vi "PanelWizard_Facade.vi"(0 "Data In":T6, 2 "Display State In":T2={"DisplayStyle"=enum."3D Style", "LaunchType"=enum."LaunchHDV", "UserVIPath"=path "", "Button Text"="", "UseDefaultButtonText?"=TRUE, "Run User VI?"=TRUE, "CommandLine"="", "StandardInput"="", "Working Directory"=path ""}, 3 "Container State":T5) -> (6 "Data Out":T6, 7 "Display State Out":T2={"DisplayStyle"=enum."3D Style", "LaunchType"=enum."LaunchHDV", "UserVIPath"=path "", "Button Text"="", "UseDefaultButtonText?"=TRUE, "Run User VI?"=TRUE, "CommandLine"="", "StandardInput"="", "Working Directory"=path ""}, 8 "Action":T1)   [LabVIEW 2012, in "PanelWizard.xctl"]
uses:
  PanelWizard.xctl
  PanelWizard_Data.ctl
  <vilib>/_xctls/Container State.ctl
  PanelWizard_State.ctl
  PanelWizard_DisplayType.ctl
  PanelWizard_LaunchOptions.ctl
  <vilib>/_xctls/Action.ctl
  <vilib>/_xctls/XControlSupport.lvlib
  <vilib>/lvdsc/NI_DSC.lvlib
panel:
  in  "RoundStyle":bool
  in  "SystemButton":bool
  in  "3dButton":bool
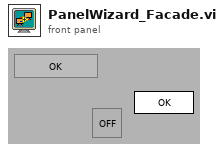
[diagram p1: front panel]
types:
  T1 = typedef "XControlSupport.lvlib/Action.ctl" = cluster{"Data Changed?":bool, "State Changed?":bool, "Action Name":string}
  T2 = typedef "PanelWizard.xctl/PanelWizard_State.ctl" = cluster{"DisplayStyle":T3, "LaunchType":T4, "UserVIPath":path, "Button Text":string, "UseDefaultButtonText?":bool, "Run User VI?":bool, "CommandLine":string, "StandardInput":string, "Working Directory":path}
  T3 = typedef "PanelWizard.xctl/PanelWizard_DisplayType.ctl" = enum16{"3D Style", "LabVIEW Classic Style", "System Style"}
  T4 = typedef "PanelWizard.xctl/PanelWizard_LaunchOptions.ctl" = enum16{"LaunchHDV", "LaunchSVMonitor", "LaunchUserVI", "Run command line"}
  T5 = typedef "XControlSupport.lvlib/Container State.ctl" = cluster{"Indicator?":bool, "Run Mode?":bool, " Refnum":refnum<vi>}
  T6 = typedef "PanelWizard.xctl/PanelWizard_Data.ctl" = bool
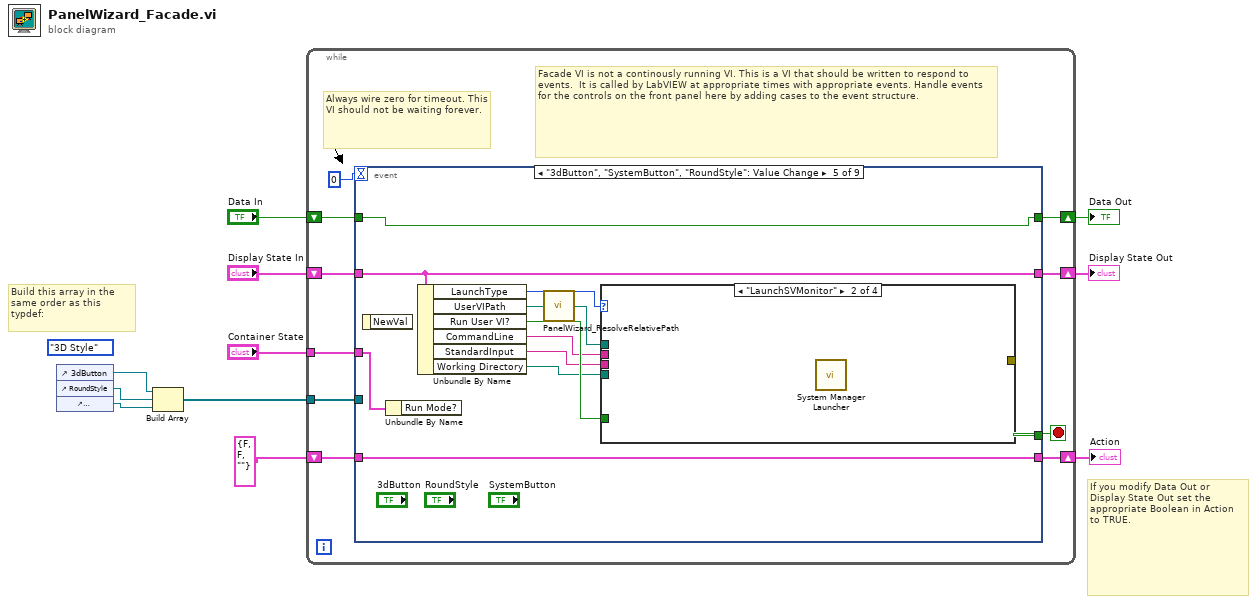
[diagram p0: block diagram]
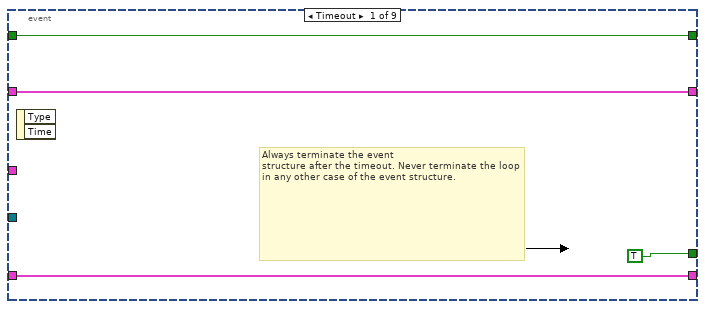
[diagram p2: hidden frame]
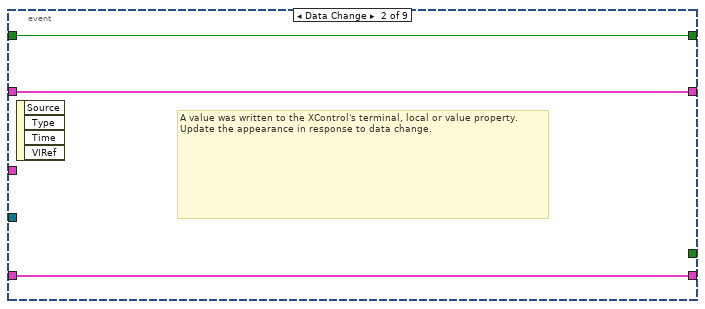
[diagram p3: hidden frame]
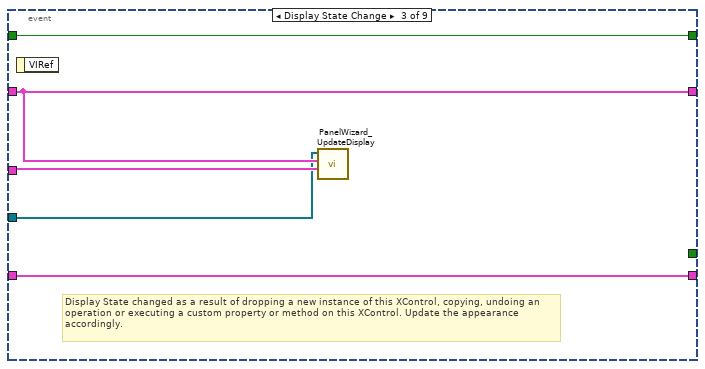
[diagram p4: hidden frame]
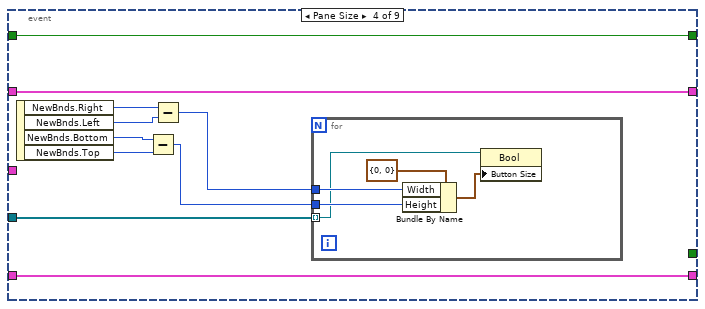
[diagram p5: hidden frame]
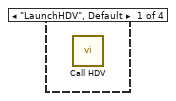
[diagram p6: hidden frame]
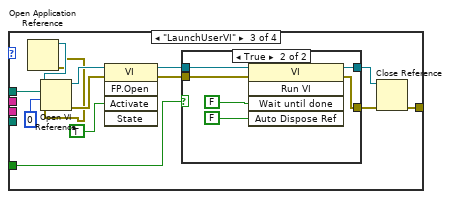
[diagram p7: hidden frame]
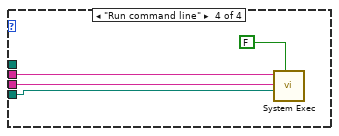
[diagram p9: hidden frame]
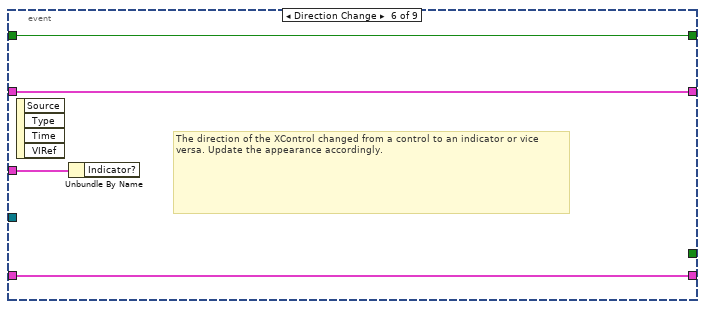
[diagram p10: hidden frame]
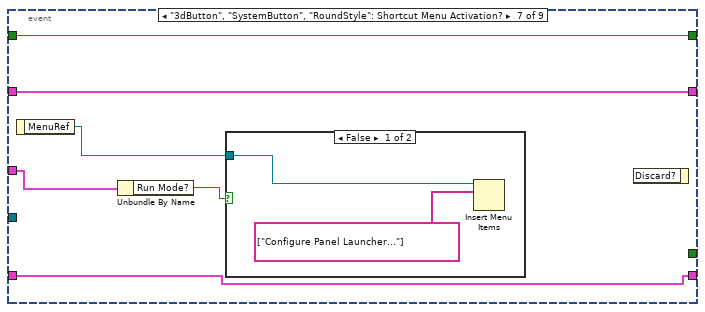
[diagram p11: hidden frame]
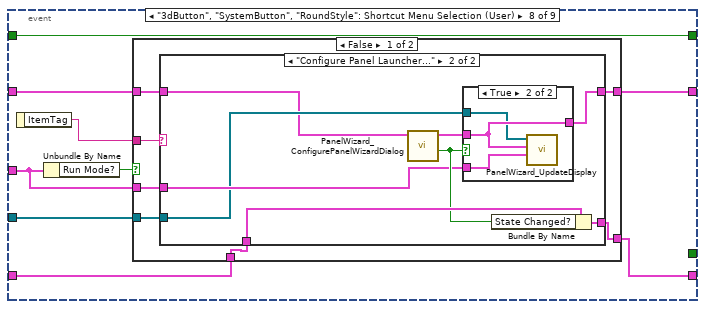
[diagram p13: hidden frame]
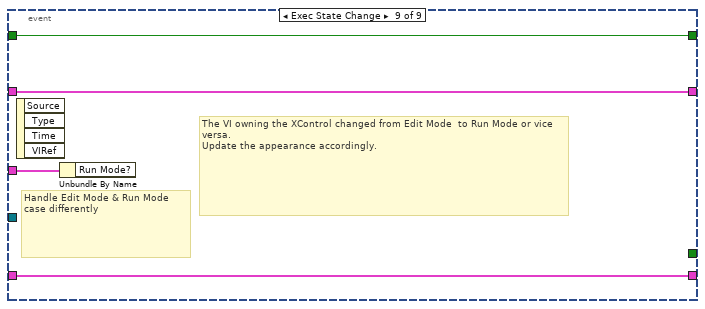
[diagram p17: hidden frame]
diagram:
  (unwired) PanelWizard_DisplayType."3D Style" ("PanelWizard_DisplayTypes")
  # "Build this array in the same order as this typdef:"
  # "If you modify Data Out or\nDisplay State Out set the\nappropriate Boolean in Action\nto TRUE."
  n1 = control-ref of="3dButton"() -> (w4:refnum<vi>)
  n2 = control-ref of="RoundStyle"() -> (w3:refnum<vi>)
  n3 = control-ref of="SystemButton"() -> (w2:refnum<vi>)
  n4 = Build Array(w4, w3, w2) -> (w1:refnum<vi>[])
  n5 = while {
    shift-right: [w20] -> w8
    shift-left: "Display State In" -> [w21]
    tunnel: "Container State" -> [w17]
    shift-right: [w15] -> w11
    shift-left: "Data In" -> [w16]
    shift-right: [w13] -> w6
    shift-left: T1 {"Data Changed?"=FALSE, "State Changed?"=FALSE, "Action Name"=""} ("Action") -> [w14]
    tunnel: w1 -> [w12]
    stop <- w19 stop-if-true
    # "Facade VI is not a continously running VI. This is a VI that should be written to respond to events.  It is called by LabVIEW at appropriate times with appropriate events. Handle events for the controls on the front panel here by adding cases to the event structure."
    # "Always wire zero for timeout. This\nVI should not be waiting forever."
    n6 = event shown="[4] \"3dButton\", \"SystemButton\", \"RoundStyle\": Value Change" {
      selector: _ -> [_ _ _ _ _ _ _ _ _]
      dyn-events: _ -> [_ _ _ _ _ _ _ _ _]
      timeout: 0 -> [_ _ _ _ _ _ _ _ _]
      tunnel: w21 -> [w23 w27 w30 w35 w57 w87 w91 w103 w131]
      tunnel: [w23 w27 w30 w35 w57 w87 w91 w102 w131] -> w20
      tunnel: [TRUE _ _ _ _ _ _ _ _] -> w19
      tunnel: w17 -> [_ _ w31 _ w55 w88 w92 w97 w132]
      tunnel: w16 -> [w22 w28 w33 w36 w56 w86 w89 w105 w130]
      tunnel: [w22 w28 w33 w36 w56 w86 w89 w105 w130] -> w15
      tunnel: [w24 w26 w32 w43 w58 w85 w90 w100 w129] -> w13
      tunnel: w14 -> [w24 w26 w32 w43 w58 w85 w90 w101 w129]
      tunnel: w12 -> [_ _ w29 w34 _ _ _ w98 _]
      event Timeout {
        # "Always terminate the event\nstructure after the timeout. Never terminate the loop in any other case of the event structure."
        n7 = event-data() -> ()  [unwired: 1 in, 2 out]
      }
      event Data Change {
        # "A value was written to the XControl's terminal, local or value property.\nUpdate the appearance in response to data change."
        n8 = event-data() -> ()  [unwired: 1 in, 4 out]
      }
      event Display State Change {
        # "Display State changed as a result of dropping a new instance of this XControl, copying, undoing an operation or executing a custom property or method on this XControl. Update the appearance accordingly."
        n9 = event-data() -> ()  [unwired: 1 in, 1 out]
        n10 = call "PanelWizard_UpdateDisplay.vi"("Container State"=w31, "Display State In"=w30, "Button Refs"=w29) -> ()  [unwired: 9 in]
      }
      event Pane Size {
        n11 = event-data() -> ("NewBnds.Right"=w42:i16, "NewBnds.Left"=w41:i16, "NewBnds.Bottom"=w40:i16, "NewBnds.Top"=w39:i16)  [unwired: 1 in]
        n12 = Subtract(x=w40, y=w39) -> (x-y=w37:i16)
        n13 = Subtract(x=w42, y=w41) -> (x-y=w38:i16)
        n14 = for {
          tunnel: w38 -> [w47]
          tunnel: w37 -> [w46]
          tunnel: w34 -> [w44] mode=indexing
          n15 = Bundle By Name(cluster=cluster{"Width":u32, "Height":u32} {"Width"=0, "Height"=0} ("Button Size"), "Width"=w47, "Height"=w46) -> (w45:cluster{"Width":u32, "Height":u32})
          n16 = property class="Bool"(reference=w44, "Button Size"=w45) -> ()  [unwired: 1 in, 2 out]
        }
      }
      event "3dButton", "SystemButton", "RoundStyle": Value Change {
        n17 = event-data() -> ()  [unwired: 1 in, 1 out]
        n18 = Unbundle By Name(w55) -> ()  [unwired: 1 out]
        n19 = Unbundle By Name(w57) -> ("LaunchType"=w59:T4, "UserVIPath"=w50:path, "Run User VI?"=w54:bool, "CommandLine"=w53:string, "StandardInput"=w52:string, "Working Directory"=w51:path)
        n20 = call "PanelWizard_ResolveRelativePath.vi"("Relative Path"=w50) -> ("Absolute  Path"=w49:path)
        n21 = case shown="\"LaunchSVMonitor\"" w59 {
          tunnel: w49 -> [_ _ w72 _]
          tunnel: [_ _ w68 _] -> _
          tunnel: w54 -> [_ _ w62 _]
          tunnel: w53 -> [_ _ _ w83]
          tunnel: w52 -> [_ _ _ w82]
          tunnel: w51 -> [_ _ _ w81]
          frame "LaunchHDV", Default {
            n22 = call <vilib>:"Call HDV.vi"() -> ()  [unwired: 14 in, 2 out]
          }
          frame "LaunchSVMonitor" {
            n23 = call "System Manager Launcher.vi"() -> ()  [unwired: 2 in]
          }
          frame "LaunchUserVI" {
            n24 = Open Application Reference() -> (0:w60:errorcluster, 3:w61:refnum<vi>)  [unwired: 4 in]
            n25 = Open VI Reference(application reference (local)=w61, vi path=w72, options=0, error in (no error)=w60) -> (vi reference=w67:refnum<vi>, error out=w64:errorcluster)  [unwired: 2 in]
            n26 = invoke class="VI" method="FP.Open"(reference=w67, error in=w64, "Activate"=TRUE ("Activate?")) -> (reference out=w66:refnum<vi>, error out=w65:errorcluster)  [unwired: 2 in, 3 out]
            n27 = case shown="True" w62 {
              tunnel: [w74 w80] -> w70
              tunnel: [w73 w79] -> w69
              tunnel: w66 -> [w74 w78]
              tunnel: w65 -> [w73 w77]
              frame False {
              }
              frame True {
                n28 = invoke class="VI" method="Run VI"(reference=w78, error in=w77, "Wait until done"=FALSE ("Wait Until Done"), "Auto Dispose Ref"=FALSE ("Wait Until Done")) -> (reference out=w80:refnum<vi>, error out=w79:errorcluster)  [unwired: 1 in, 3 out]
              }
            }
            n29 = Close Reference(reference=w70, error in (no error)=w69) -> (error out=w68:errorcluster)
          }
          frame "Run command line" {
            n30 = call <vilib>:"System Exec.vi"("wait until completion? (T)"=FALSE, "working directory"=w81, "standard input"=w82, "command line"=w83) -> ()  [unwired: 4 in, 4 out]
          }
        }
      }
      event Direction Change {
        # "The direction of the XControl changed from a control to an indicator or vice versa. Update the appearance accordingly."
        n31 = event-data() -> ()  [unwired: 1 in, 4 out]
        n32 = Unbundle By Name(w88) -> ()  [unwired: 1 out]
      }
      event "3dButton", "SystemButton", "RoundStyle": Shortcut Menu Activation? {
        n33 = event-data() -> ("MenuRef"=w93:refnum<k9>)  [unwired: 1 in]
        n34 = Unbundle By Name(w92) -> ("Run Mode?"=w94:bool)
        n35 = case shown="False" w94 {
          tunnel: w93 -> [w96 _]
          frame False {
            n36 = Insert Menu Items(8:string[] ["Configure Panel Launcher..."] ("item names"), 9:w96) -> ()  [unwired: 4 in, 3 out]
          }
          frame True {
          }
        }
        n37 = event-data() -> ()  [unwired: 2 in, 1 out]
      }
      event "3dButton", "SystemButton", "RoundStyle": Shortcut Menu Selection (User) {
        n38 = event-data() -> ("ItemTag"=w99:string)  [unwired: 1 in]
        n39 = Unbundle By Name(w97) -> ("Run Mode?"=w104:bool)
        n40 = case shown="False" w104 {
          tunnel: w99 -> [w112 _]
          tunnel: w103 -> [w111 w128]
          tunnel: [w108 w128] -> w102
          tunnel: w101 -> [w109 w127]
          tunnel: [w110 w127] -> w100
          tunnel: w97 -> [w107 _]
          tunnel: w98 -> [w106 _]
          frame False {
            n41 = case shown="\"Configure Panel Launcher...\"" w112 {
              tunnel: w111 -> [w114 w115]
              tunnel: [w113 w122] -> w110
              tunnel: w109 -> [w113 w121]
              tunnel: [w114 w118] -> w108
              tunnel: w107 -> [_ w117]
              tunnel: w106 -> [_ w116]
              frame Default {
              }
              frame "Configure Panel Launcher..." {
                n42 = call "PanelWizard_ConfigurePanelWizardDialog.vi"("Display State"=w115) -> ("Updated?"=w120:bool, "Display State Out"=w119:T2)  [unwired: 9 in]
                n43 = case shown="True" w120 {
                  tunnel: w119 -> [w123 w126]
                  tunnel: [w123 w126] -> w118
                  tunnel: w117 -> [_ w125]
                  tunnel: w116 -> [_ w124]
                  frame False {
                  }
                  frame True {
                    n44 = call "PanelWizard_UpdateDisplay.vi"("Container State"=w125, "Display State In"=w126, "Button Refs"=w124) -> ()  [unwired: 9 in]
                  }
                }
                n45 = Bundle By Name(cluster=w121, "State Changed?"=w120) -> (w122:T1)
              }
            }
          }
          frame True {
          }
        }
      }
      event Exec State Change {
        # "The VI owning the XControl changed from Edit Mode  to Run Mode or vice versa.\nUpdate the appearance accordingly."
        # "Handle Edit Mode & Run Mode\ncase differently"
        n46 = event-data() -> ()  [unwired: 1 in, 4 out]
        n47 = Unbundle By Name(w132) -> ()  [unwired: 1 out]
      }
    }
  }
  "Display State Out" <- w8
  "Data Out" <- w11
  "Action" <- w6
